vi "DACConv.vi"(1 "Maximum":dbl format="%.1f", 2 "Minimum":dbl format="%.1f", 3 "Input":dbl format="%.1f", 4 "Type":enum16{"Counts to Voltage", "Voltage to Counts"}(ring)) -> (0 "Output":dbl format="%.1f")   [LabVIEW 2014]
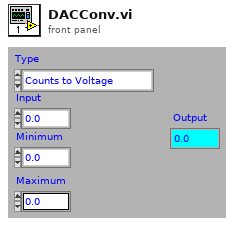
[diagram p1: front panel]
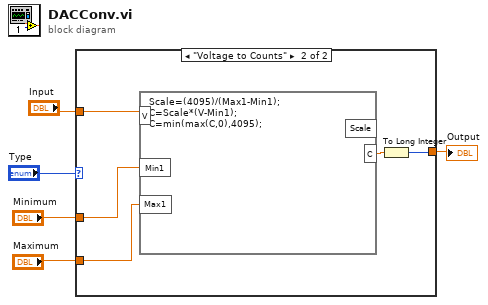
[diagram p0: block diagram]
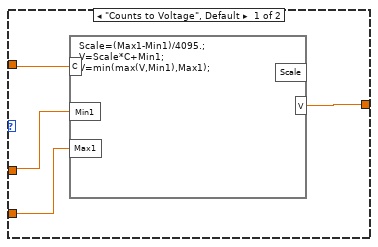
[diagram p2: hidden frame]
diagram:
  n1 = case shown="\"Voltage to Counts\"" "Type" {
    tunnel: "Input" -> [w6 w14]
    tunnel: [w7 w10] -> w3
    tunnel: "Minimum" -> [w9 w13]
    tunnel: "Maximum" -> [w8 w12]
    frame "Counts to Voltage", Default {
      n2 = formula code="Scale=(Max1-Min1)/4095.;\nV=Scale*C+Min1;\nV=min(max(V,Min1),Max1);"("C"=w6, "Min1"=w9, "Max1"=w8) -> ("V"=w7:dbl)  [unwired: 1 out]
    }
    frame "Voltage to Counts" {
      n3 = formula code="Scale=(4095)/(Max1-Min1);\nC=Scale*(V-Min1);\nC=min(max(C,0),4095);"("V"=w14, "Min1"=w13, "Max1"=w12) -> ("C"=w11:dbl)  [unwired: 1 out]
      n4 = To Long Integer(number=w11) -> (32bit integer=w10:i32)
    }
  }
  "Output" <- w3
